vi "Dequeue.vi"(6 "EnqueueType (QMH)":T2, 7 "DequeueType (PreviewQueue)":T1, 8 "error in (no error)":errorcluster, 10 "timeout in ms (100)":i32=100, 11 "Queue Array Reference In":refnum<queue>[](array[refnum])) -> (0 "error out":errorcluster, 1 "Message Data":variant, 2 "Message":string, 3 "MessageQueue":refnum<queue>, 5 "Queue Array Reference Out":refnum<queue>[](array[refnum]))   [LabVIEW 2018, in "ScopeModule.lvlib"]
uses:
  ScopeModule.lvlib
  PublicAPI/Arguments/Messages/clMessage.ctl
  ScopePlugins/TypeDefs/QueueNames.ctl
  ScopePlugins/TypeDefs/DequeueTypes.ctl
  ScopePlugins/ScopePlugins.lvlib
panel:
  out "timed out?":bool
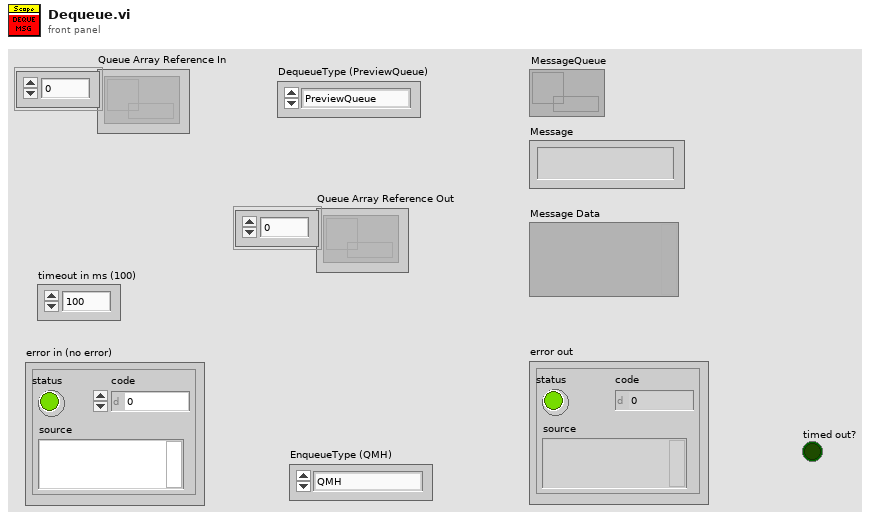
[diagram p1: front panel]
types:
  T1 = typedef "ScopePlugins.lvlib/DequeueTypes.ctl" = enum16{"PreviewQueue", "Dequeue"}
  T2 = typedef "ScopePlugins.lvlib/QueueNames.ctl" = enum16{"QMH", "Class ", "MA"}
  T3 = typedef "ScopeModule.lvlib/clMessage.ctl" = cluster{"Message":string, "Message Data":variant}
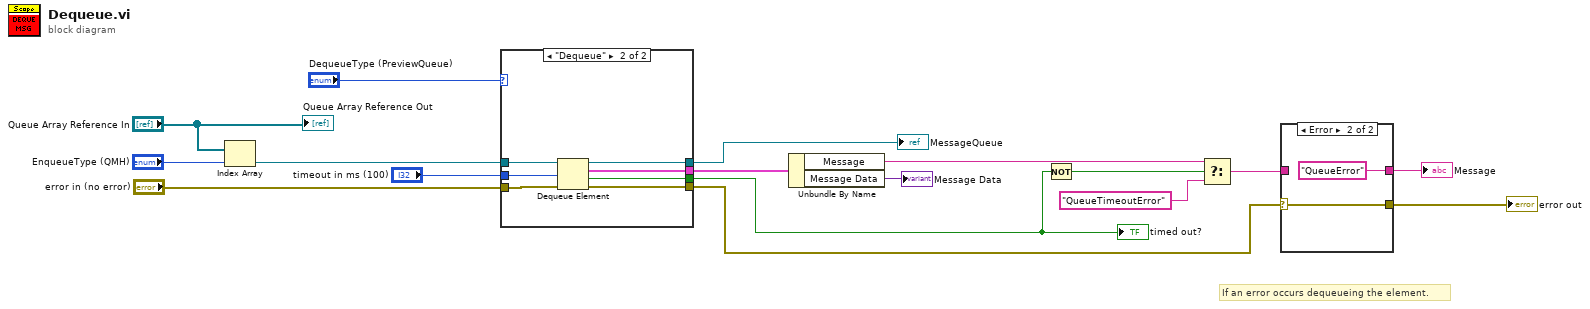
[diagram p0: block diagram]
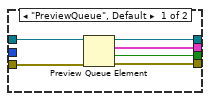
[diagram p3: hidden frame]
diagram:
  # "If an error occurs dequeueing the element."
  n1 = Index Array(array="Queue Array Reference In", index="EnqueueType (QMH)") -> (element=w2:refnum<queue>)
  n2 = case shown="\"Dequeue\"" "DequeueType (PreviewQueue)" {
    tunnel: [w20 w30] -> w9
    tunnel: [w19 w29] -> w17
    tunnel: [w21 w28] -> w15
    tunnel: "error in (no error)" -> [w23 w27]
    tunnel: w2 -> [w22 w26]
    tunnel: [w18 w25] -> w5
    tunnel: "timeout in ms (100)" -> [_ w24]
    frame "PreviewQueue", Default {
      n3 = Preview Queue Element(queue=w22, error in (no error)=w23) -> (queue out=w21:refnum<queue>, element=w19:T3, timed out?=w18:bool, error out=w20:errorcluster)  [unwired: 1 in]
    }
    frame "Dequeue" {
      n4 = Dequeue Element(queue=w26, timeout in ms (-1)=w24, error in (no error)=w27) -> (queue out=w28:refnum<queue>, element=w29:T3, timed out?=w25:bool, error out=w30:errorcluster)
    }
  }
  "MessageQueue" <- w15
  "timed out?" <- w5
  n5 = Unbundle By Name(w17) -> ("Message"=w6:string, "Message Data"=→"Message Data":variant)
  n6 = Not(x=w5) -> (.not. x?=w12:bool)
  n7 = Select(t=w6, s=w12, f="QueueTimeoutError" ("Message")) -> (s? t:f=w11:string)
  n8 = case shown="Error" w9 {
    selector: w9 -> [w31 w33]
    tunnel: w11 -> [w32 _]
    tunnel: [w32 "QueueError" ("Message")] -> w7
    tunnel: [w31 w33] -> w8
    frame No Error {
    }
    frame Error {
    }
  }
  "error out" <- w8
  "Message" <- w7
  "Queue Array Reference Out" <- "Queue Array Reference In"
